vi "ExSimpleSPD.vi"() -> ()   [LabVIEW 2010]
panel:
  in  "stop":bool
  in  "Detecotr (only available for NCL)":u32=1 min=1 max=3 step=1
  in  "Num of Reads to average":u32=1 min=1 step=1
  in  "Gain Range":u32 max=4 step=1
  in  "Integraion / Exposure ms":dbl=1.0 min=1.0 step=1.0 format="%.2f"
  in  "Detector Type":u32=1 min=1 max=3 step=1
  in  "Bi Polar Enable":bool
  in  "High Volts":dbl format="%.2f"
  in  "High Volts Enable":bool
  out "Detector Type":u32
  out "Bi Polar":bool
  out "Gain Value":dbl format="%.2f"
  out "Gain Range":dbl format="%.2f"
  out "Integraion time ms":dbl format="%.2f"
  out "HV Status":bool
  out "HV Volts":dbl format="%.2f"
  out "Get Ave Rds":u32
  out "reserve 2":u32
  out "reserve 1":u32
  out "Voltage":dbl format="%.2f"
  out "error out":errorcluster
  in  "error in (no error)":errorcluster
  # "ExSimpleSPD.vi: this example shows how to control\none single point Detector. The values are set on the\n left and the results are display on the right.\nIn the center is the live reading of the SPT."
  # "1 :  Current\n 2 :  Voltage\n 3 :  Photon Counting"
  # "Minimum is 1.0 ms\nPractical minimum 10.0 ms\nTypical 100.0 ms\nmaximum is 65 sec (65535ms)"
  # "0 : 1x\n1 :  2x\n2 :  4x\n3 : 50x\n4 : 200x"
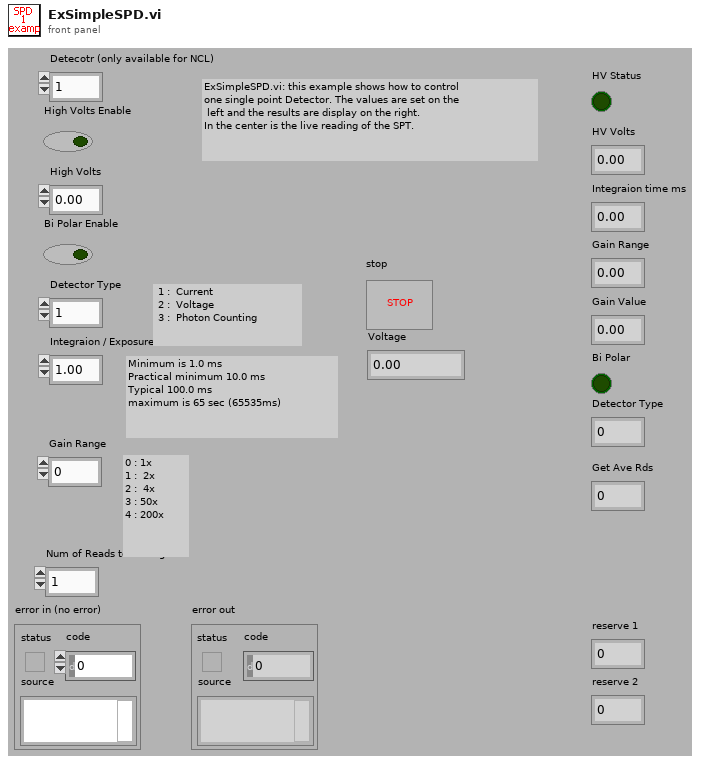
[diagram p1: front panel]
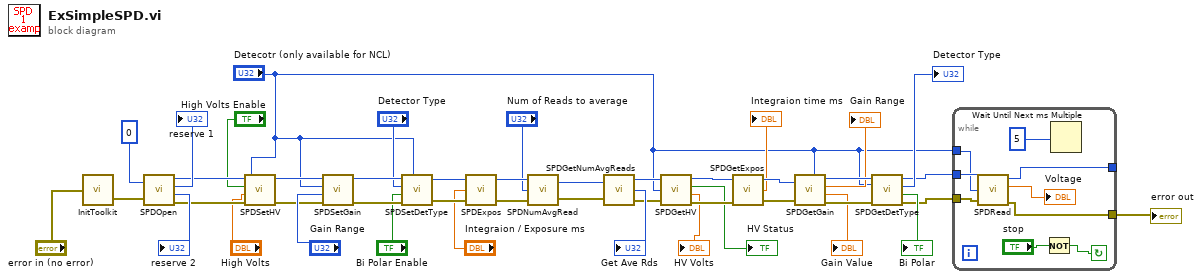
[diagram p0: block diagram]
diagram:
  n1 = call <userlib>:"InitToolkit.vi"("error in"="error in (no error)") -> ("error out"=w1:errorcluster)
  n2 = call <userlib>:"SPDOpen.vi"("Device ID"=0, "error in (no error)"=w1) -> ("SPD Handle"=w23:u32, "reserved 1"=→"reserve 1":u32, "reserved 2"=→"reserve 2":u32, "error out"=w24:errorcluster)
  n3 = call <userlib>:"SPDSetHV.vi"("SPD Handle"=w23, "HV enable/disable"="High Volts Enable", "Volts"="High Volts", "error in (no error)"=w24, "SPD Number"="Detecotr (only available for NCL)") -> ("SPD Handle"=w18:u32, "error out"=w19:errorcluster)
  n4 = call <userlib>:"SPDSetGain.vi"("error in (no error)"=w19, "Gain Range"="Gain Range", "Detector Number"="Detecotr (only available for NCL)", "SPD Handle"=w18) -> ("error out"=w17:errorcluster, "SPD Handle"=w16:u32)
  n5 = call <userlib>:"SPDSetDetType.vi"("SPD Handle"=w16, "Detector Type"="Detector Type", "BiPolar switch"="Bi Polar Enable", "error in (no error)"=w17, "SPD Number"="Detecotr (only available for NCL)") -> ("SPD Handle"=w12:u32, "error out"=w13:errorcluster)
  n6 = call <userlib>:"SPDExpos.vi"("error in (no error)"=w13, "Integration Time (ms)"="Integraion / Exposure ms", "SPD Handle"=w12) -> ("error out"=w10:errorcluster, "SPD Handle"=w9:u32)
  n7 = call <userlib>:"SPDNumAvgRead.vi"("error in (no error)"=w10, "Number to average Reads"="Num of Reads to average", "SPD Handle"=w9) -> ("error out"=w8:errorcluster, "SPD Handle"=w7:u32)
  n8 = call <userlib>:"SPDGetNumAvgReads.vi"("SPD Handle"=w7, "error in (no error)"=w8) -> ("SPD Handle"=w25:u32, "Number of Averages"=→"Get Ave Rds":u32, "error out"=w26:errorcluster)
  n9 = call <userlib>:"SPDGetHV.vi"("SPD Handle"=w25, "Detector Number"="Detecotr (only available for NCL)", "error in (no error)"=w26) -> ("SPD Handle"=w36:u32, "HV Status (ON/OFF)"=→"HV Status":bool, "HV Volts"=→"HV Volts":dbl, "error out"=w39:errorcluster)
  n10 = call <userlib>:"SPDGetExpos.vi"("error in (no error)"=w39, "SPD Handle"=w36) -> ("error out"=w38:errorcluster, "Integration time in ms"=→"Integraion time ms":dbl, "SPD Handle"=w35:u32)  [unwired: 1 in]
  n11 = call <userlib>:"SPDGetGain.vi"("Detector Number"="Detecotr (only available for NCL)", "error in (no error)"=w38, "SPD Handle"=w35) -> ("error out"=w37:errorcluster, "Gain value"=→"Gain Value":dbl, "Gain Range"=→"Gain Range":dbl, "SPD Handle"=w34:u32)
  n12 = call <userlib>:"SPDGetDetType.vi"("SPD Handle"=w34, "SPD Number"="Detecotr (only available for NCL)", "error in (no error)"=w37) -> ("SPD Handle"=w4:u32, "Detector Type"=→"Detector Type":u32, "BiPolar state"=→"Bi Polar":bool, "error out"=w5:errorcluster)
  n13 = while {
    tunnel: w5 -> [w53]
    tunnel: w4 -> [w52]
    tunnel: "Detecotr (only available for NCL)" -> [w51]
    tunnel: [w49] -> _
    tunnel: [w48] -> w2
    stop <- w46 continue-if-true
    n14 = call <userlib>:"SPDRead.vi"("SPD Handle"=w52, "Detector Number"=w51, "error in (no error)"=w53) -> ("SPD Handle"=w49:u32, "SPD Value"=→"Voltage":dbl, "error out"=w48:errorcluster)  [unwired: 1 out]
    n15 = Not(x="stop") -> (.not. x?=w46:bool)
    n16 = Wait Until Next ms Multiple(millisecond multiple=5) -> ()  [unwired: 1 out]
  }
  "error out" <- w2
